vi "Preset Builder.vi"(8 "Column Header":string[](array[string]), 9 "Input Table":string[][](table)) -> (1 "Exit Indicator":bool, 2 "Output Table":string[][](table))   [LabVIEW 2020]
uses:
  Preset Query Enum.ctl
  Search 2D Array (String).vi
panel:
  in  "Tab Control":enum32{"Main", "Controls"}(tab)
  in  "FilterReset":bool
  in  "Filter Button":bool
  in  "Filter":string
  in  "Clear Table":bool
  in  "Copy Whole Table":bool
  in  "Select an ECS file":path
  in  "Preset Menu":u16(ring) items=["None", "1Hz", "26J", "Amp2, Clunker In", "Amp3-17J", "Amp3-30J-FrogFoilIn", "Amp3-8J-CapExit", "Amp3-MegaAttenuator", "CW", "Cameras free run - BELLA", "Cameras triggered - BELLA", "Cameras triggered - DataLogging", "Diode", "FW-Safe", "JetIn", "LaserTableExposure1Hz", "MagSpecSimulateBoff", "MagSpecSimulateBon", "NewmarkStageTest", "Pulsed", "Pulsed Alignment", "SMFiber-In", "SMFiber-Out", "SingleShot", "Staging-Jet in (4.5mm lower than laser)", "Staging-SMF fiber-in", "dev_simcam_2", "dev_simcam_3", "developer_test_1", "try stage"]
  in  "Current Table":bool
  in  "RESET":bool
  in  "EXIT":bool
  in  "Source":i32[](listbox)
  in  "Selected Rows":i32[](listbox)
  in  "EXIT 2":bool
  in  "Source Copy":i32[](listbox)
  # "How to use :\n\nDrag the rows you want to keep to the selected rows table. \n\nUse CTRL or SHIFT to select multiple values at once.\n\nRight-Click > Delete Row to delete a row in the Selected Rows Table"
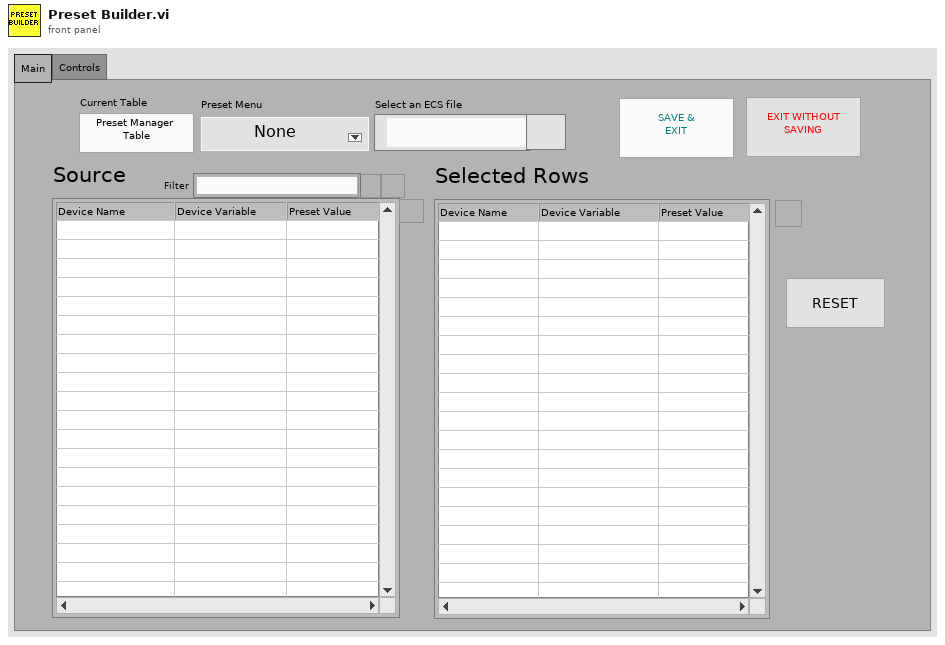
[diagram p1: front panel]
types:
  T1 = typedef "Preset Query Enum.ctl" = enum16{"Get Locations", "Get all IPs and MACs", "Get classes", "Get expt variables to set at scanstart for particular device", "Get expt devices and variables with start values", "Get expt devices and variables (with data to get)", "Get expt devices with data to get", "Get Expt devices and GUIs", "Get all devices basic properties", "Get Virtual Devices Core Info", "Get Expt names", "Get experiment basic properties", "Get experiment alarm variables", "Get MC Ports", "Get device network comm port", "Get devicetype lvclass path", "Get basic device properties", "Get Init Order", "Get all setable variables of a device", "Get device variable aliases", "Get force values of all settable variables", "Get all variables of a devicetype", "Get all variables of a device", "Get plotter details", "Get Saved Scans", "Get Scan Info", "GetGeneralGUIs", "Get expt for plotter", "Get plotter IDs from expt", "Get all devices", "Get all Virtual Devices", "Get all aliases", "Get variable and device info for Virtual Device", "GetItemLocatorIP", "Get IPs for GUIs", "Get DeviceType from Device", "GetLocalPortRange", "GetDevicePresetVariables", "Get Device Configuration", "GetAllPresetNames", "GetAllConfigurationNames", "GetPresetDeviceNames", "GetDeviceAliases", "GetDevicesOfClass"}
  T2 = typedef "LVPoint32TypeDef.ctl" = cluster{"Horizontal":i32, "Vertical":i32}
  T3 = typedef "LVRowAndColumnTypeDef.ctl" = cluster{"Row":i32, "Column":i32}
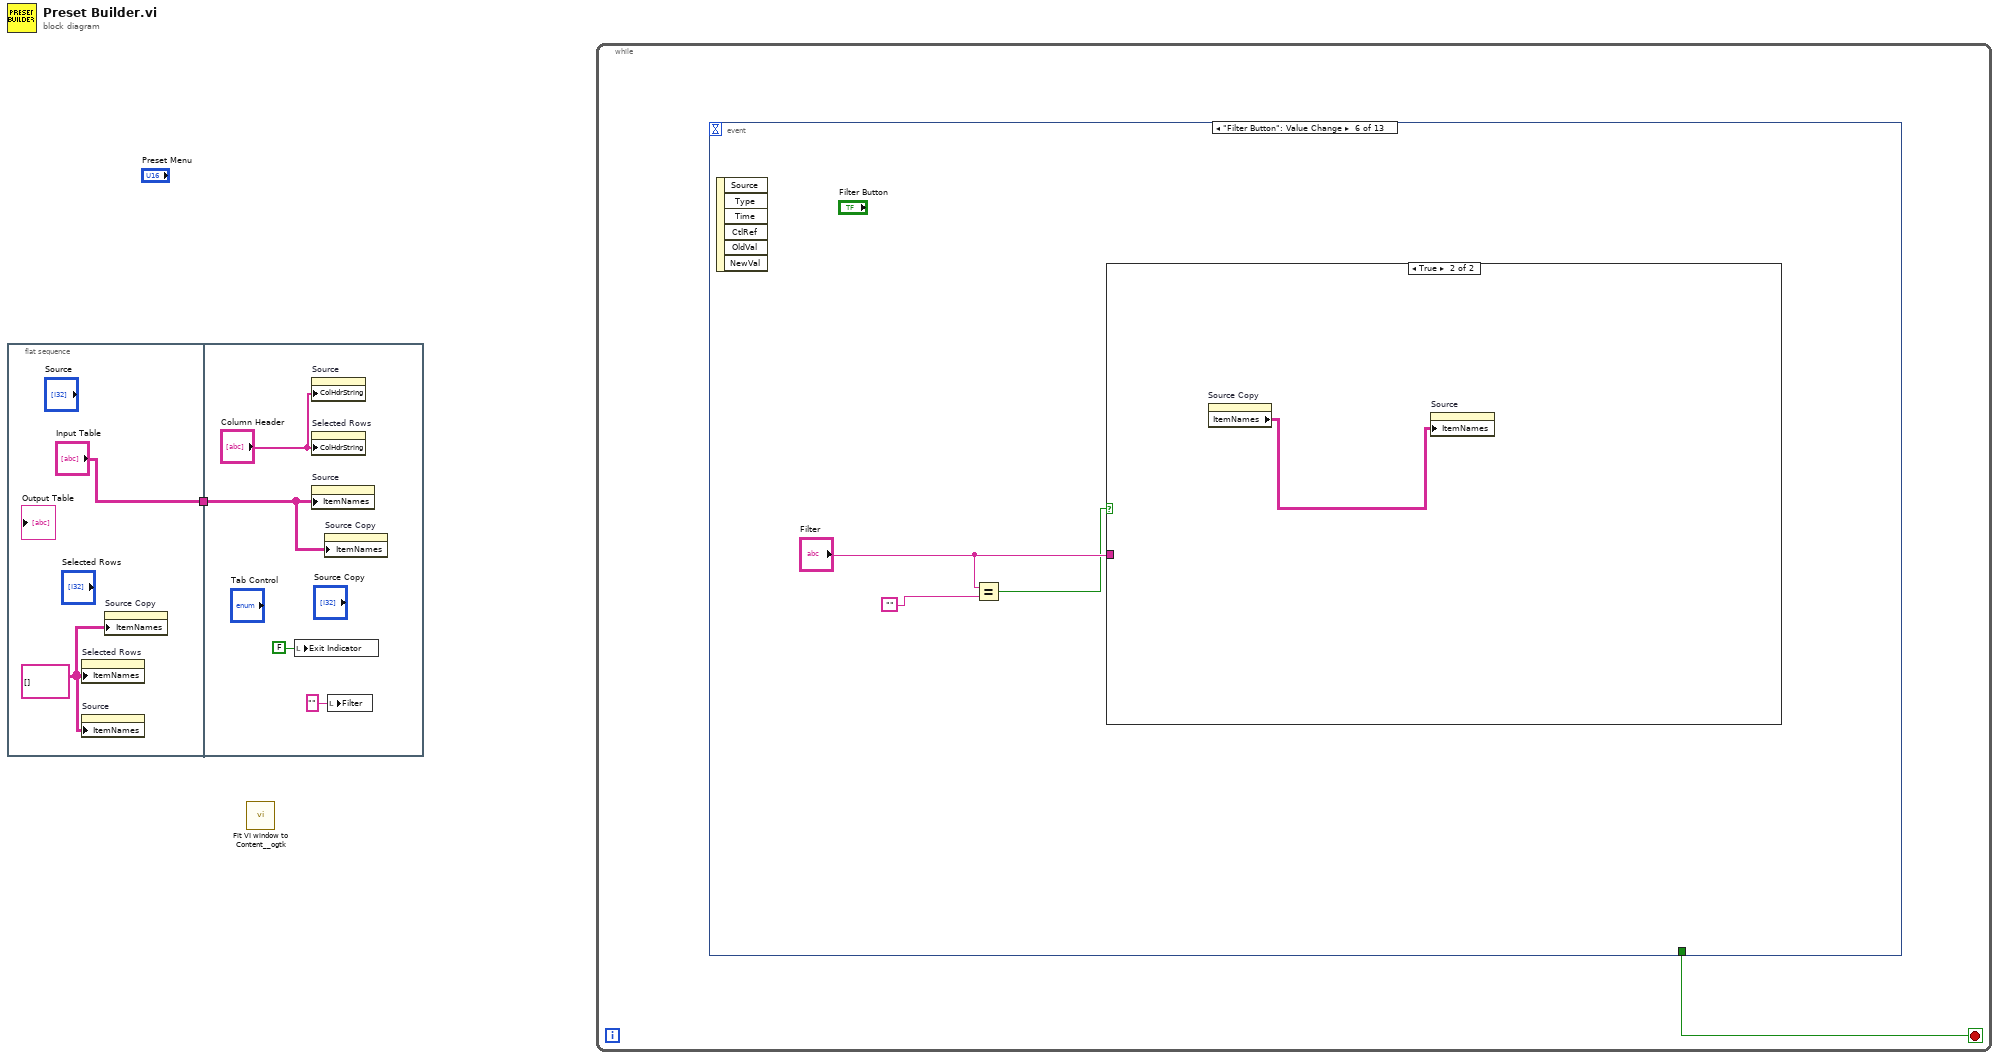
[diagram p0: block diagram]
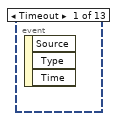
[diagram p2: hidden frame]
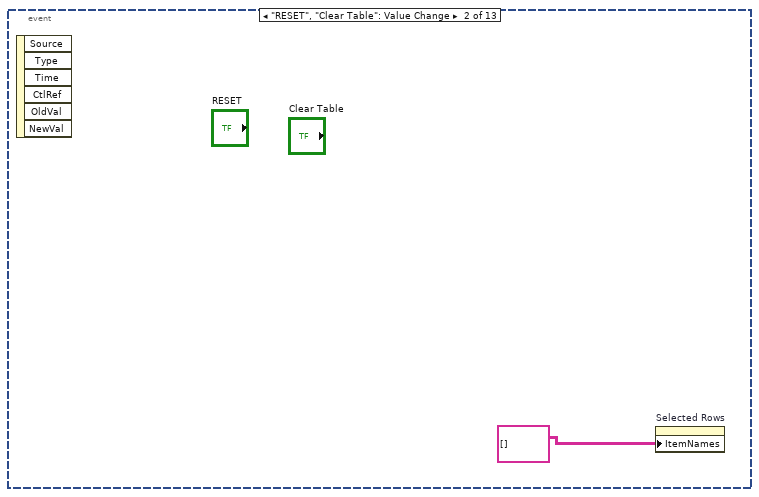
[diagram p3: hidden frame]
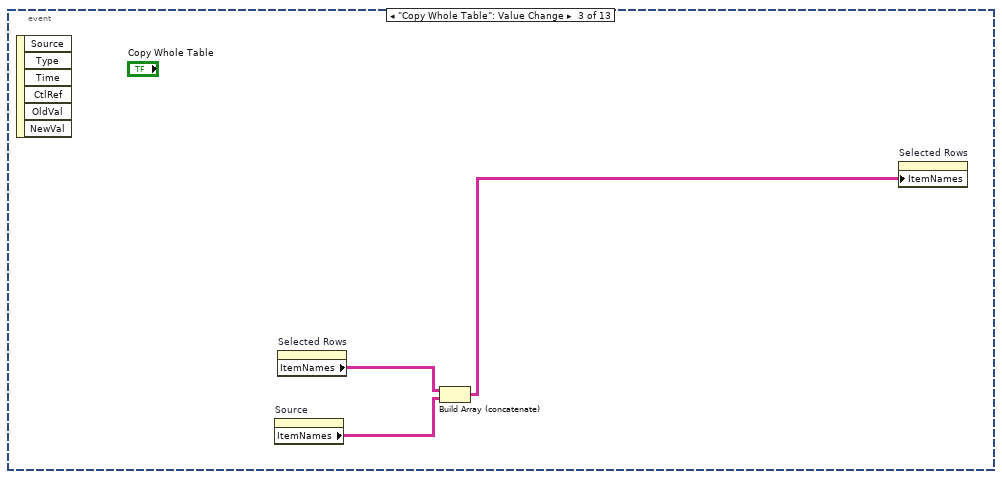
[diagram p4: hidden frame]
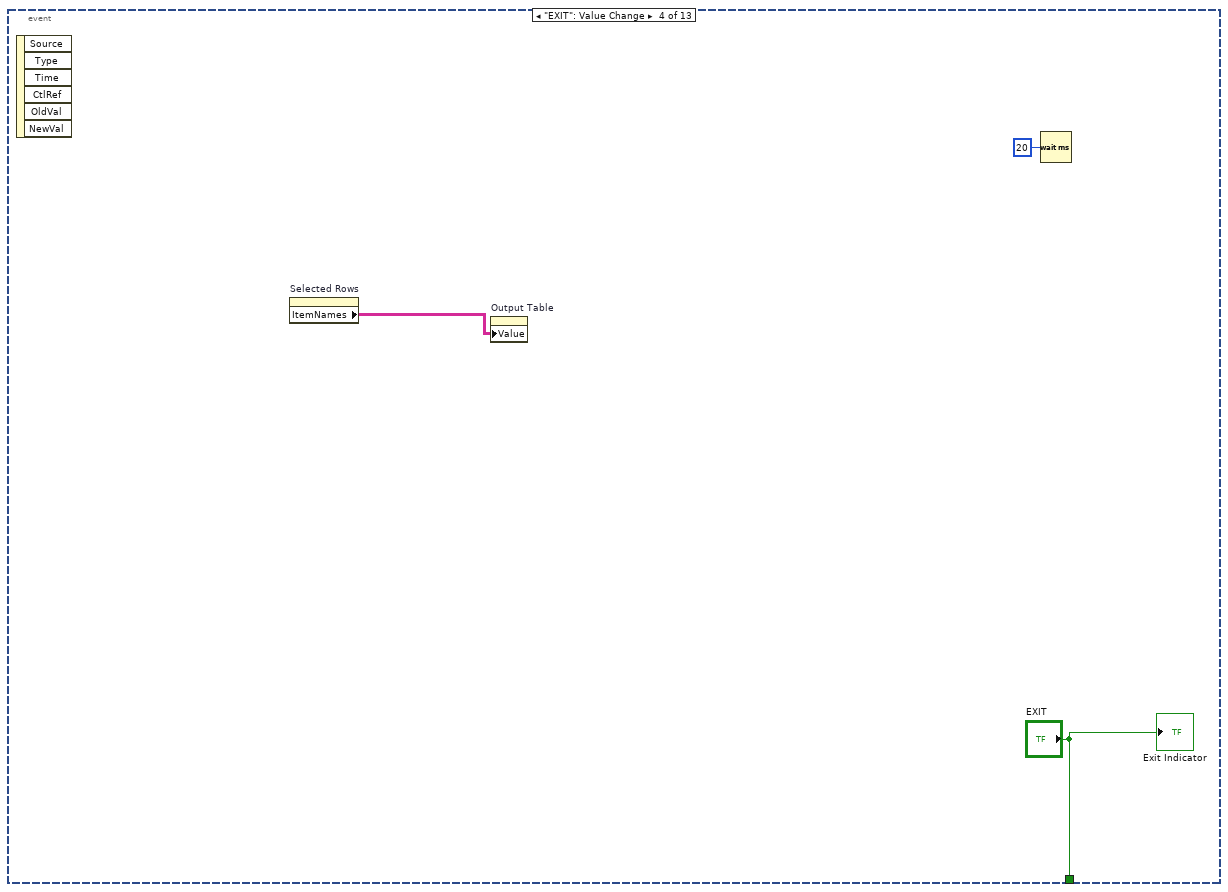
[diagram p5: hidden frame]
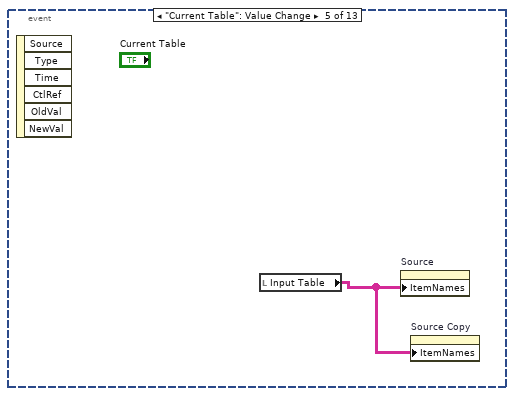
[diagram p6: hidden frame]
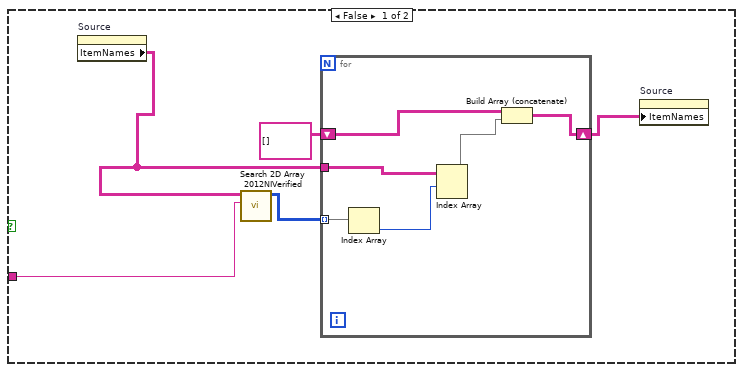
[diagram p7: hidden frame]
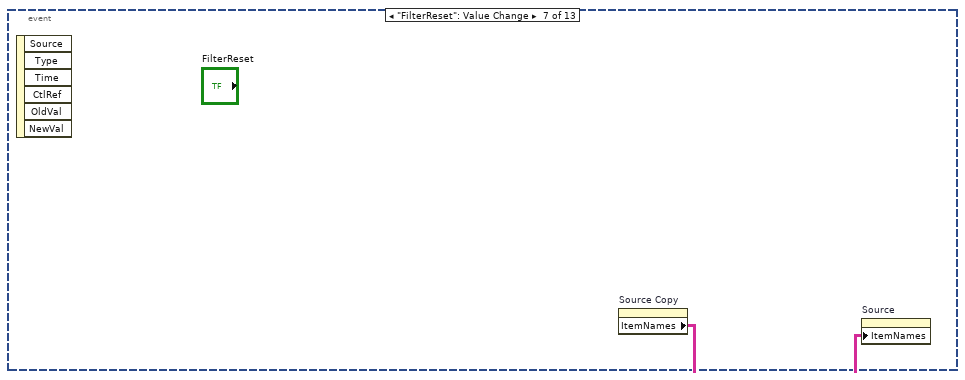
[diagram p8: hidden frame]
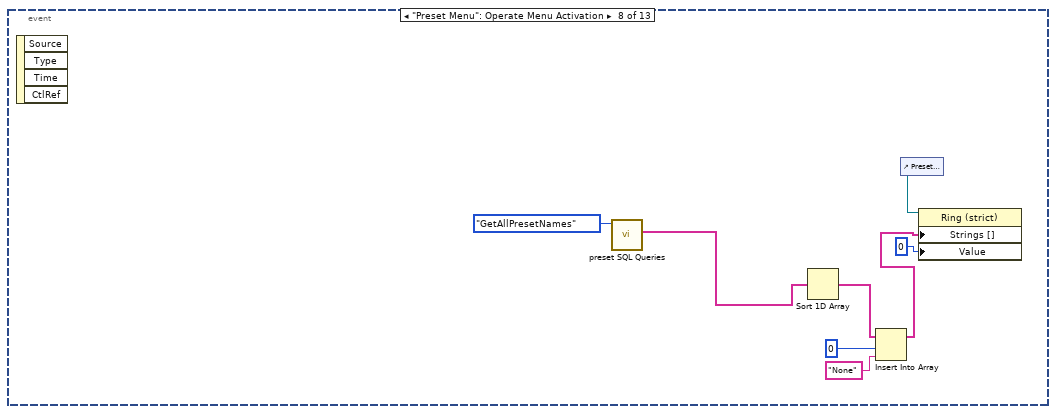
[diagram p9: hidden frame]
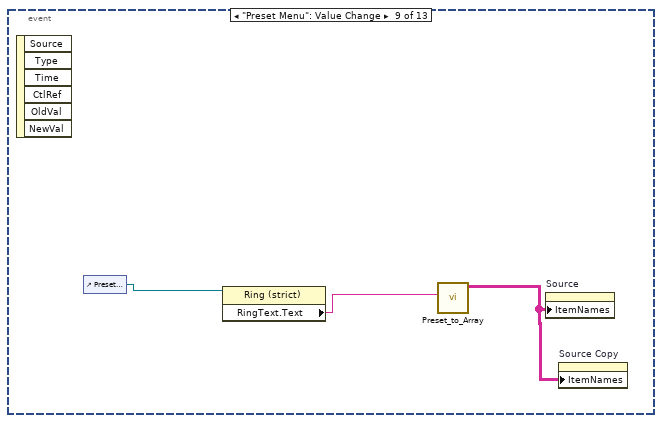
[diagram p10: hidden frame]
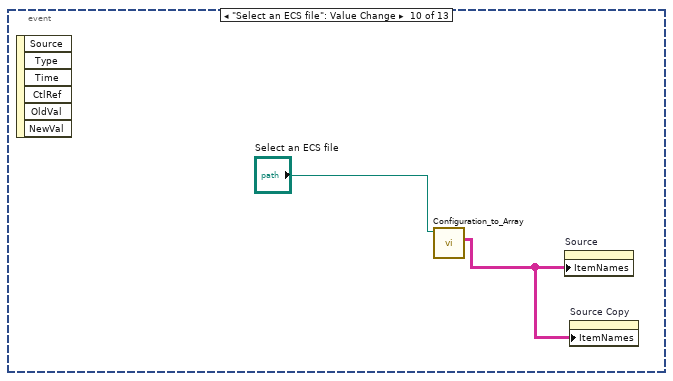
[diagram p11: hidden frame]
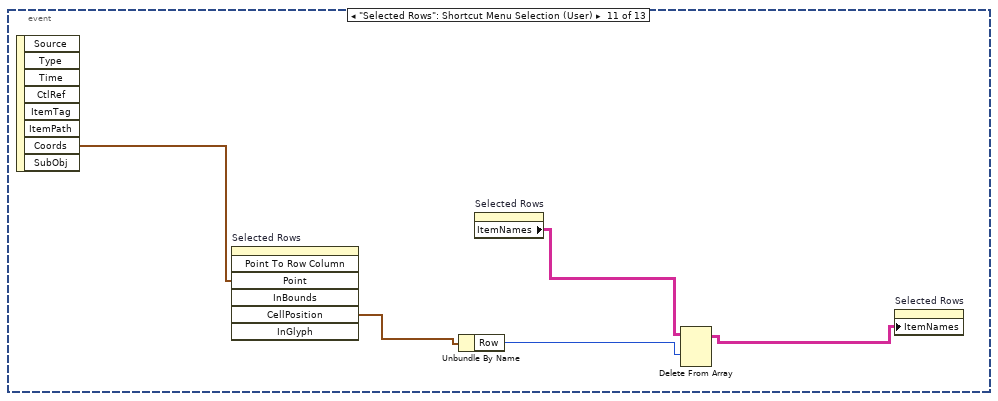
[diagram p12: hidden frame]
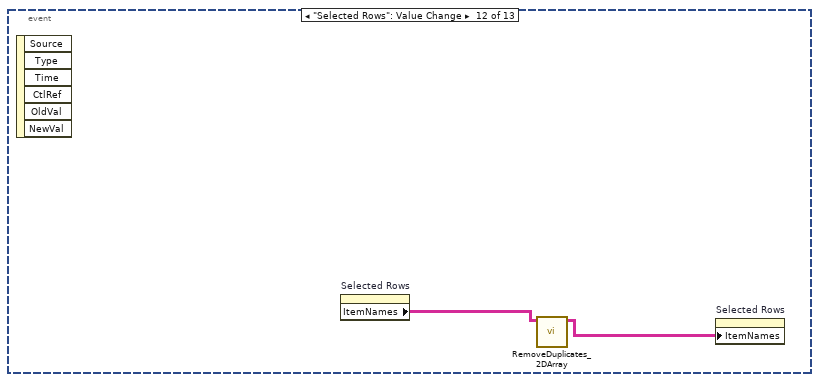
[diagram p13: hidden frame]
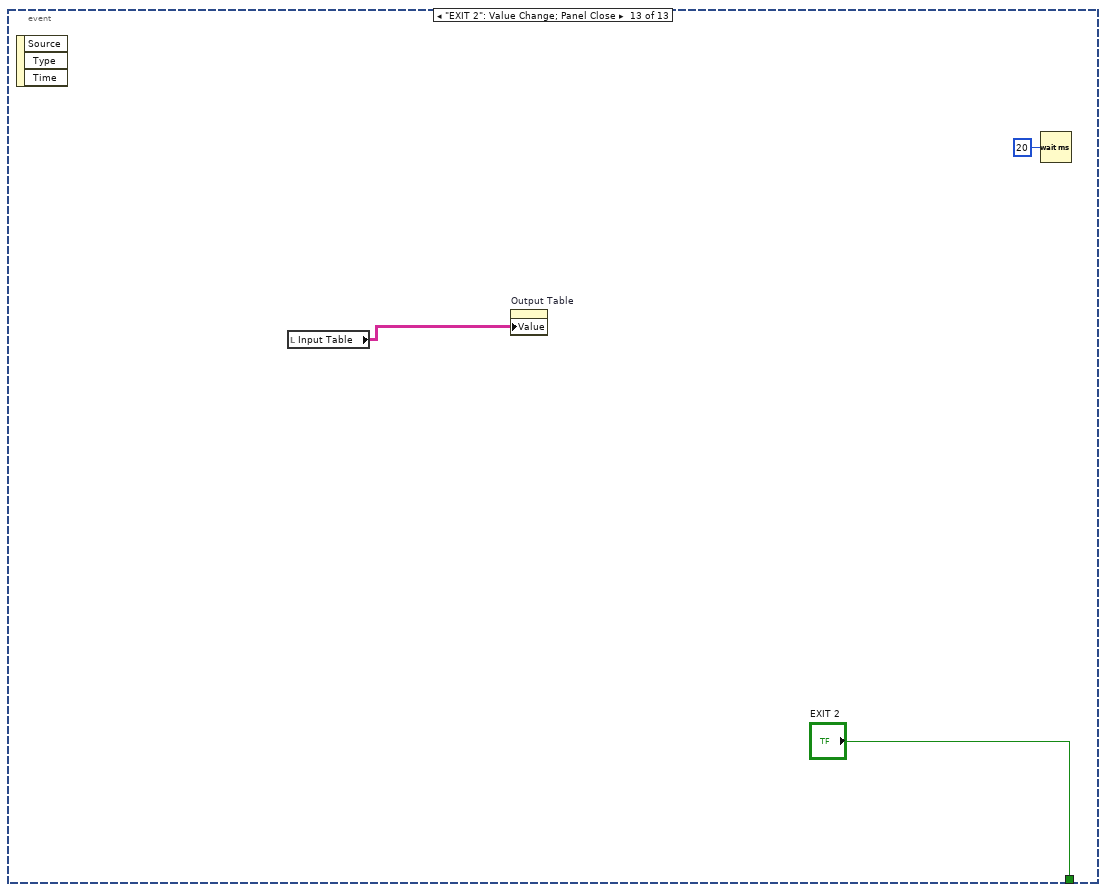
[diagram p14: hidden frame]
diagram:
  n1 = flat-sequence {
    tunnel: ["Input Table"] -> w1
    tunnel: w1 -> [w5]
    frame #0 {
      w2 = string[][] [] ("Table Control 2")
      n2 = property on="Selected Rows" class="MCListbox (strict)"("ItemNames"=w2) -> ()  [unwired: 2 in, 2 out]
      n3 = property on="Source" class="MCListbox (strict)"("ItemNames"=w2) -> ()  [unwired: 2 in, 2 out]
      n4 = property on="Source Copy" class="MCListbox (strict)"("ItemNames"=w2) -> ()  [unwired: 2 in, 2 out]
    }
    frame #1 {
      n5 = local write "Exit Indicator"(FALSE ("Exit Indicator")) -> ()
      n6 = property on="Source" class="MCListbox (strict)"("ColHdrString"="Column Header") -> ()  [unwired: 2 in, 2 out]
      n7 = property on="Selected Rows" class="MCListbox (strict)"("ColHdrString"="Column Header") -> ()  [unwired: 2 in, 2 out]
      n8 = property on="Source" class="MCListbox (strict)"("ItemNames"=w5) -> ()  [unwired: 2 in, 2 out]
      n9 = property on="Source Copy" class="MCListbox (strict)"("ItemNames"=w5) -> ()  [unwired: 2 in, 2 out]
      n10 = local write "Filter"("" ("Filter")) -> ()
    }
  }
  n11 = call <userlib>:"Fit VI window to Content__ogtk.vi"() -> ()  [unwired: 6 in, 2 out]
  n12 = while {
    stop <- w8 stop-if-true
    n13 = event shown="[5] \"Filter Button\": Value Change" {
      selector: _ -> [_ _ _ _ _ _ _ _ _ _ _ _ _]
      dyn-events: _ -> [_ _ _ _ _ _ _ _ _ _ _ _ _]
      timeout: _ -> [_ _ _ _ _ _ _ _ _ _ _ _ _]
      tunnel: [_ _ _ "EXIT" _ _ _ _ _ _ _ _ "EXIT 2"] -> w8
      event Timeout {
        n14 = event-data() -> ()  [unwired: 1 in, 3 out]
      }
      event "RESET", "Clear Table": Value Change {
        n15 = event-data() -> ()  [unwired: 1 in, 6 out]
        n16 = property on="Selected Rows" class="MCListbox (strict)"("ItemNames"=string[][] [] ("Table Control 2")) -> ()  [unwired: 2 in, 2 out]
      }
      event "Copy Whole Table": Value Change {
        n17 = event-data() -> ()  [unwired: 1 in, 6 out]
        n18 = property on="Source" class="MCListbox (strict)"() -> ("ItemNames"=w11:string[][])  [unwired: 2 in, 2 out]
        n19 = property on="Selected Rows" class="MCListbox (strict)"() -> ("ItemNames"=w12:string[][])  [unwired: 2 in, 2 out]
        n20 = Build Array (concatenate)(w12, w11) -> (w10:string[][])
        n21 = property on="Selected Rows" class="MCListbox (strict)"("ItemNames"=w10) -> ()  [unwired: 2 in, 2 out]
      }
      event "EXIT": Value Change {
        n22 = event-data() -> ()  [unwired: 1 in, 6 out]
        n23 = property on="Selected Rows" class="MCListbox (strict)"() -> ("ItemNames"=w13:string[][])  [unwired: 2 in, 2 out]
        n24 = property on="Output Table" class="Tbl (strict)"("Value"=w13) -> ()  [unwired: 2 in, 2 out]
        n25 = Wait (ms)(milliseconds to wait=u32 20) -> ()  [unwired: 1 out]
        "Exit Indicator" <- "EXIT"
      }
      event "Current Table": Value Change {
        n26 = event-data() -> ()  [unwired: 1 in, 6 out]
        n27 = local read "Input Table"() -> (w16:string[][])
        n28 = property on="Source" class="MCListbox (strict)"("ItemNames"=w16) -> ()  [unwired: 2 in, 2 out]
        n29 = property on="Source Copy" class="MCListbox (strict)"("ItemNames"=w16) -> ()  [unwired: 2 in, 2 out]
      }
      event "Filter Button": Value Change {
        n30 = event-data() -> ()  [unwired: 1 in, 6 out]
        n31 = Equal?(x="Filter", y="") -> (x = y?=w17:bool)
        n32 = case shown="True" w17 {
          tunnel: "Filter" -> [w24 _]
          frame False {
            n33 = property on="Source" class="MCListbox (strict)"() -> ("ItemNames"=w20:string[][])  [unwired: 2 in, 2 out]
            n34 = call-poly "Search 2D Array 2012NIVerified.vi"("Element"=w24, "Array"=w20) -> ("Locations"=w23:i32[][])  [unwired: 9 in]
            n35 = for {
              tunnel: w23 -> [w30] mode=indexing
              shift-right: [w26] -> w22
              shift-left: string[][] [] -> [w27]
              tunnel: w20 -> [w25]
              n36 = Index Array(array=w30) -> (element=w29:i32)  [unwired: 1 in]
              n37 = Index Array(array=w25, index (row)=w29) -> (element=w28:string[])  [unwired: 1 in]
              n38 = Build Array (concatenate)(w27, w28) -> (w26:string[][])
            }
            n39 = property on="Source" class="MCListbox (strict)"("ItemNames"=w22) -> ()  [unwired: 2 in, 2 out]
          }
          frame True {
            n40 = property on="Source Copy" class="MCListbox (strict)"() -> ("ItemNames"=w31:string[][])  [unwired: 2 in, 2 out]
            n41 = property on="Source" class="MCListbox (strict)"("ItemNames"=w31) -> ()  [unwired: 2 in, 2 out]
          }
        }
      }
      event "FilterReset": Value Change {
        n42 = event-data() -> ()  [unwired: 1 in, 6 out]
        n43 = property on="Source Copy" class="MCListbox (strict)"() -> ("ItemNames"=w32:string[][])  [unwired: 2 in, 2 out]
        n44 = property on="Source" class="MCListbox (strict)"("ItemNames"=w32) -> ()  [unwired: 2 in, 2 out]
      }
      event "Preset Menu": Operate Menu Activation {
        n45 = event-data() -> ()  [unwired: 1 in, 4 out]
        n46 = call "preset SQL Queries.vi"("Preset Query"=Preset_Query_Enum."GetAllPresetNames") -> ("1st column 1st data"=w37:string[])  [unwired: 8 in, 2 out]
        n47 = Sort 1D Array(array=w37) -> (sorted array=w34:string[])
        n48 = Insert Into Array(array=w34, index=0, new element="None" ("new element/subarray")) -> (w33:string[])
        n49 = control-ref of="Preset Menu"() -> (w38:refnum<vi>)
        n50 = property on="Property Node" class="Ring (strict)"(reference=w38, "Strings []"=w33, "Value"=0 ("index")) -> ()  [unwired: 1 in, 2 out]
      }
      event "Preset Menu": Value Change {
        n51 = event-data() -> ()  [unwired: 1 in, 6 out]
        n52 = control-ref of="Preset Menu"() -> (w43:refnum<vi>)
        n53 = property on="Property Node" class="Ring (strict)"(reference=w43) -> ("RingText.Text"=w42:string)  [unwired: 1 in, 2 out]
        n54 = call "Preset_to_Array.vi"("Preset Name"=w42) -> ("Preset Table"=w41:string[][])  [unwired: 9 in, 1 out]
        n55 = property on="Source" class="MCListbox (strict)"("ItemNames"=w41) -> ()  [unwired: 2 in, 2 out]
        n56 = property on="Source Copy" class="MCListbox (strict)"("ItemNames"=w41) -> ()  [unwired: 2 in, 2 out]
      }
      event "Select an ECS file": Value Change {
        n57 = event-data() -> ()  [unwired: 1 in, 6 out]
        n58 = call "Configuration_to_Array.vi"("file (use dialog)"="Select an ECS file") -> ("Table Control"=w44:string[][])  [unwired: 10 in]
        n59 = property on="Source" class="MCListbox (strict)"("ItemNames"=w44) -> ()  [unwired: 2 in, 2 out]
        n60 = property on="Source Copy" class="MCListbox (strict)"("ItemNames"=w44) -> ()  [unwired: 2 in, 2 out]
      }
      event "Selected Rows": Shortcut Menu Selection (User) {
        n61 = event-data() -> ("Coords"=w50:T2)  [unwired: 1 in, 7 out]
        n62 = invoke on="Selected Rows" class="MCListbox (strict)" method="Point To Row Column"("Point"=w50) -> ("CellPosition"=w49:T3)  [unwired: 6 in, 6 out]
        n63 = Unbundle By Name(w49) -> ("Row"=w48:i32)
        n64 = property on="Selected Rows" class="MCListbox (strict)"() -> ("ItemNames"=w47:string[][])  [unwired: 2 in, 2 out]
        n65 = Delete From Array(array=w47, index (row)=w48) -> (array with subset deleted=w46:string[][])  [unwired: 2 in, 1 out]
        n66 = property on="Selected Rows" class="MCListbox (strict)"("ItemNames"=w46) -> ()  [unwired: 2 in, 2 out]
      }
      event "Selected Rows": Value Change {
        n67 = event-data() -> ()  [unwired: 1 in, 6 out]
        n68 = property on="Selected Rows" class="MCListbox (strict)"() -> ("ItemNames"=w51:string[][])  [unwired: 2 in, 2 out]
        n69 = call "RemoveDuplicates_2DArray.vi"("Input Array"=w51) -> ("Removed Duplicate Array"=w52:string[][])  [unwired: 10 in]
        n70 = property on="Selected Rows" class="MCListbox (strict)"("ItemNames"=w52) -> ()  [unwired: 2 in, 2 out]
      }
      event "EXIT 2": Value Change; Panel Close {
        n71 = event-data() -> ()  [unwired: 1 in, 3 out]
        n72 = local read "Input Table"() -> (w53:string[][])
        n73 = property on="Output Table" class="Tbl (strict)"("Value"=w53) -> ()  [unwired: 2 in, 2 out]
        n74 = Wait (ms)(milliseconds to wait=u32 20) -> ()  [unwired: 1 out]
      }
    }
  }
